vi "MENU_About.vi"() -> ()   [LabVIEW 2010]
panel:
  in  "Close":bool
  # "Software for the E-Field Mill hardware\nVersion 3.1.3"
  # "For more informations:\nhttp://www.kwos.org"
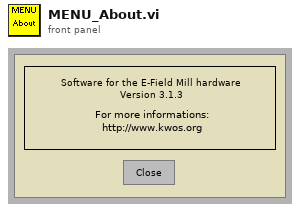
[diagram p1: front panel]
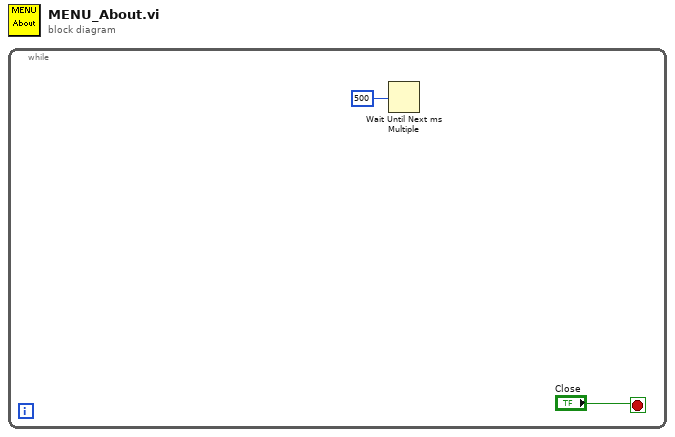
[diagram p0: block diagram]
diagram:
  n1 = while {
    stop <- "Close" stop-if-true
    n2 = Wait Until Next ms Multiple(millisecond multiple=500) -> ()  [unwired: 1 out]
  }
